vi "Start Async.vi"(8 "error in (no error)":errorcluster, 11 "gRPC Server in":refnum<class "iService.lvclass">) -> (0 "error out":errorcluster, 3 "gRPC Server out":refnum<class "iService.lvclass">)   [LabVIEW 2019, in "gRPC-servicer.lvlib" / "iService.lvclass"]
uses:
  iService.lvclass
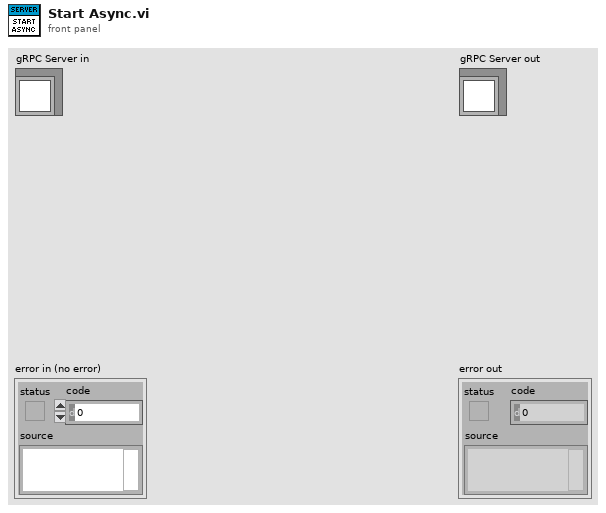
[diagram p1: front panel]
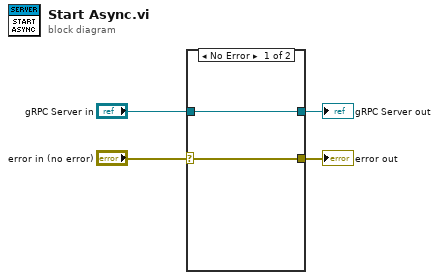
[diagram p0: block diagram]
diagram:
  n1 = case shown="No Error" "error in (no error)" {
    selector: "error in (no error)" -> [w5 w8]
    tunnel: [w5 w8] -> w3
    tunnel: [w6 w7] -> w1
    tunnel: "gRPC Server in" -> [w6 w7]
    frame No Error {
    }
    frame Error {
    }
  }
  "error out" <- w3
  "gRPC Server out" <- w1
